vi "GCMPlugin_IsSupportingItem.vi"(8 "error in (no error)":errorcluster, 9 "VI Reference":refnum<vi>, 10 "ProjectItem Refnum":refnum<vi>, 11 "_EnumEditor in":refnum<class "_EnumEditor.lvclass">) -> (0 "error out":errorcluster, 2 "IsSupportingItem":bool, 3 "_EnumEditor out":refnum<class "_EnumEditor.lvclass">)   [LabVIEW 2014, in "_EnumEditor.lvclass"]
uses:
  _EnumEditor.lvclass
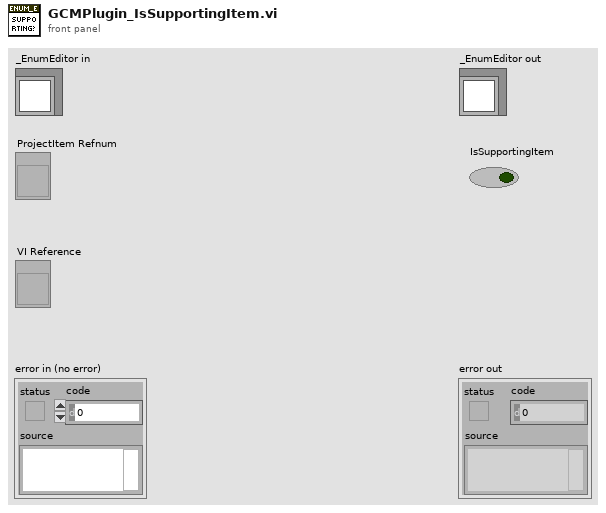
[diagram p1: front panel]
types:
  T1 = enum32{"invalid VI type", "Standard VI", "Control VI", "Global VI", "Polymorphic VI", "Configuration VI", "SubSystem", "Facade VI", "Method VI", "Statechart Diagram VI"}
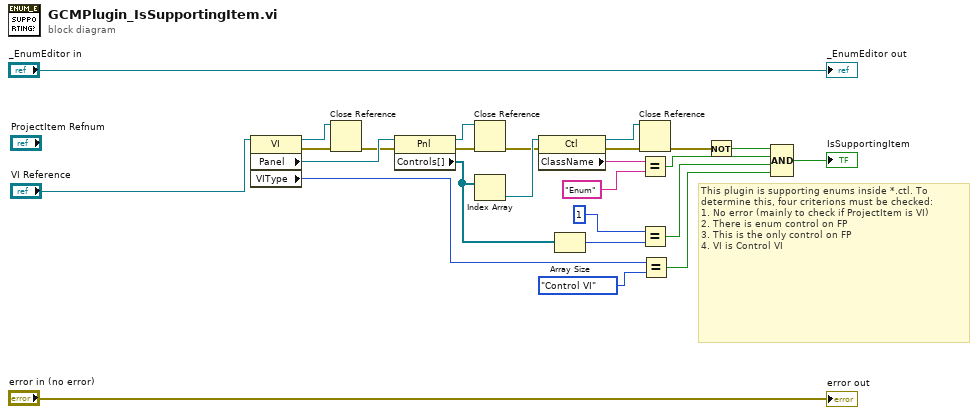
[diagram p0: block diagram]
diagram:
  # "This plugin is supporting enums inside *.ctl. To determine this, four criterions must be checked:\n1. No error (mainly to check if ProjectItem is VI)\n2. There is enum control on FP\n3. This is the only control on FP\n4. VI is Control VI"
  n1 = property class="VI"(reference="VI Reference") -> (reference out=w8:refnum<vi>, error out=w10:errorcluster, "Panel"=w24:refnum<vi>, "VIType"=w4:T1)  [unwired: 1 in]
  n2 = Close Reference(reference=w8, error in (no error)=w10) -> (error out=w9:errorcluster)
  n3 = property class="Pnl"(reference=w24, error in=w9) -> (reference out=w6:refnum<vi>, error out=w7:errorcluster, "Controls[]"=w22:refnum<vi>[])
  n4 = Close Reference(reference=w6, error in (no error)=w7) -> (error out=w5:errorcluster)
  n5 = Index Array(array=w22) -> (element=w23:refnum<vi>)  [unwired: 1 in]
  n6 = property class="Ctl"(reference=w23, error in=w5) -> (reference out=w12:refnum<vi>, error out=w17:errorcluster, "ClassName"=w19:string)
  n7 = Array Size(array=w22) -> (size(s)=w21:i32)
  n8 = Close Reference(reference=w12, error in (no error)=w17) -> (error out=w13:errorcluster)
  n9 = Equal?(x=w19, y="Enum") -> (x = y?=w16:bool)
  n10 = Equal?(x=1, y=w21) -> (x = y?=w15:bool)
  n11 = Equal?(x=w4, y=T1."Control VI") -> (x = y?=w2:bool)
  n12 = Not(x=w13) -> (.not. x?=w11:bool)
  n13 = Compound Arithmetic op=AND(w11, w16, w15, w2) -> (→"IsSupportingItem":bool)
  "error out" <- "error in (no error)"
  "_EnumEditor out" <- "_EnumEditor in"
